vi "Destroy.vi"(8 "error in (no error)":errorcluster, 11 "Console Log in":refnum<class "Console Log.lvclass">) -> (0 "error out":errorcluster, 3 "Console Log out":refnum<class "Console Log.lvclass">)   [LabVIEW 2011, in "Console Log.lvclass"]
uses:
  Console Log.lvclass
  Console Log.lvclass/Console Log.ctl
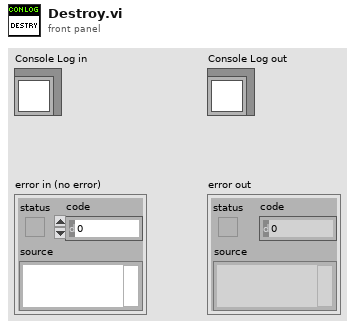
[diagram p1: front panel]
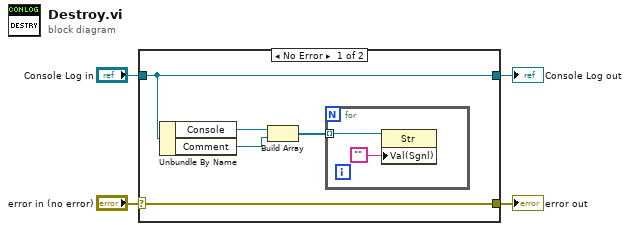
[diagram p0: block diagram]
diagram:
  n1 = case shown="No Error" "error in (no error)" {
    selector: "error in (no error)" -> [w9 w13]
    tunnel: [w9 w13] -> w3
    tunnel: [w8 w12] -> w1
    tunnel: "Console Log in" -> [w8 w12]
    frame No Error {
      n2 = Unbundle By Name(w8) -> ("Console"=w7:refnum<vi>, "Comment"=w6:refnum<vi>)
      n3 = Build Array(w7, w6) -> (w5:refnum<vi>[])
      n4 = for {
        tunnel: w5 -> [w11] mode=indexing
        n5 = property class="Str"(reference=w11, "Val(Sgnl)"="") -> ()  [unwired: 1 in, 2 out]
      }
    }
    frame Error {
    }
  }
  "error out" <- w3
  "Console Log out" <- w1
